vi "Excute.vi"(8 "error in (no error)":errorcluster, 11 "Decorator in":refnum<class "Decorator.lvclass">) -> (0 "error out":errorcluster, 3 "Decorator out":refnum<class "Decorator.lvclass">)   [LabVIEW 2014, in "Decorator.lvclass"]
uses:
  Decorator.lvclass
  Decorator.lvclass/Decorator.ctl
  Component_class/Component.lvclass
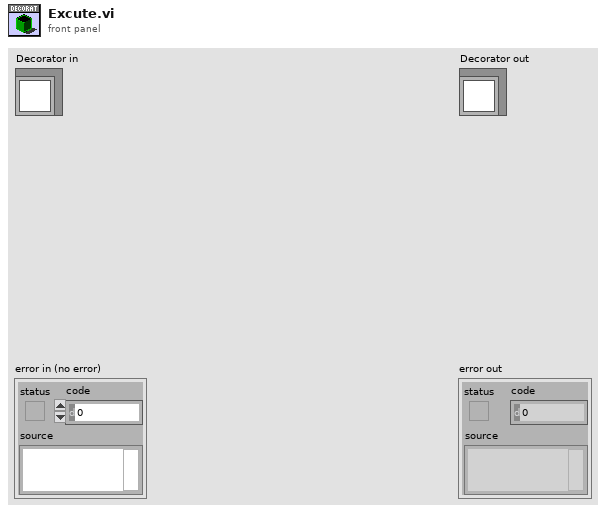
[diagram p1: front panel]
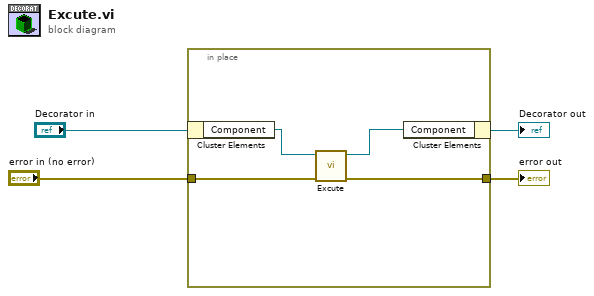
[diagram p0: block diagram]
diagram:
  n1 = in-place {
    in-place-border: "error in (no error)" -> [w6]
    in-place-border: [w5] -> w1
    n2 = in-place-cluster #1("Decorator in") -> ("Component"=w8:refnum<class "Component.lvclass">)
    n3 = call-dynamic "Excute.vi"("error in (no error)"=w6, "Component in"=w8) -> ("error out"=w5:errorcluster, "Component out"=w7:refnum<class "Component.lvclass">)  [unwired: 8 in]
    n4 = in-place-cluster #1("Component"=w7) -> (→"Decorator out":refnum<class "Decorator.lvclass">)
  }
  "error out" <- w1
